vi "Instrument.MessageFromProcess.vi"(6 "Message ID":u32, 8 "error in (no error)":errorcluster, 9 "Message.Data":variant, 10 "Message.Command":string, 11 "Instrument":refnum<class "Instrument.lvclass">) -> (0 "error out":errorcluster, 3 "Instrument out":refnum<class "Instrument.lvclass">)   [LabVIEW 2016, in "Instrument.lvclass"]
doc: "---------------------------------------------------------------\nJKI State Machine Objects™\nhttp://jki.net/state-machine-objects/\nCopyright (C) 2005-2015, JKI <info@jki.net>\nALL RIGHTS RESERVEDJKI State Machine Objects (SMO) 1.0.0.4\nJKI - JKI\nCopyright (c) 2015, JKI"
uses:
  Instrument.lvclass
  Typedefs/PublicEvents--Instrument.MessageFromProcess.ctl
  Instrument.lvclass/Instrument.ctl
panel:
  # "For instructions on how to use the JKI State Machine Objects, examples and video tutorials, visit:\nhttp://jki.net/state-machine-objects/\n\nJKI State Machine Objects™\nhttp://jki.net/state-machine-objects/\nCopyright (C) 2005-2015, JKI <info@jki.net>\nALL RIGHTS RESERVED"
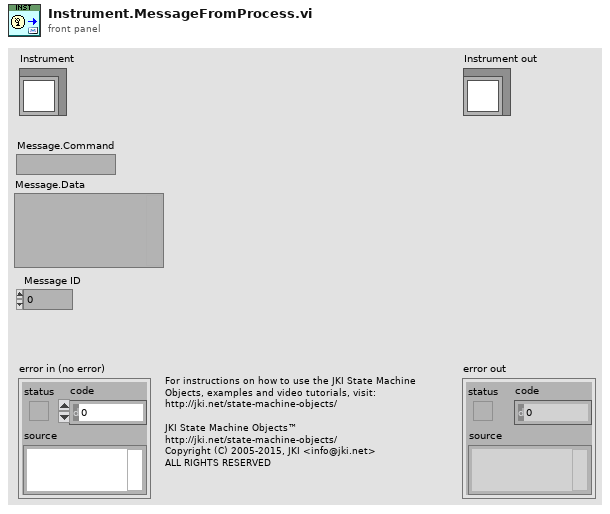
[diagram p1: front panel]
types:
  T1 = typedef "Instrument.lvclass/PublicEvents--Instrument.MessageFromProcess.ctl" = cluster{"Message":cluster{"Command":string, "Data":variant}, "Message ID":u32}
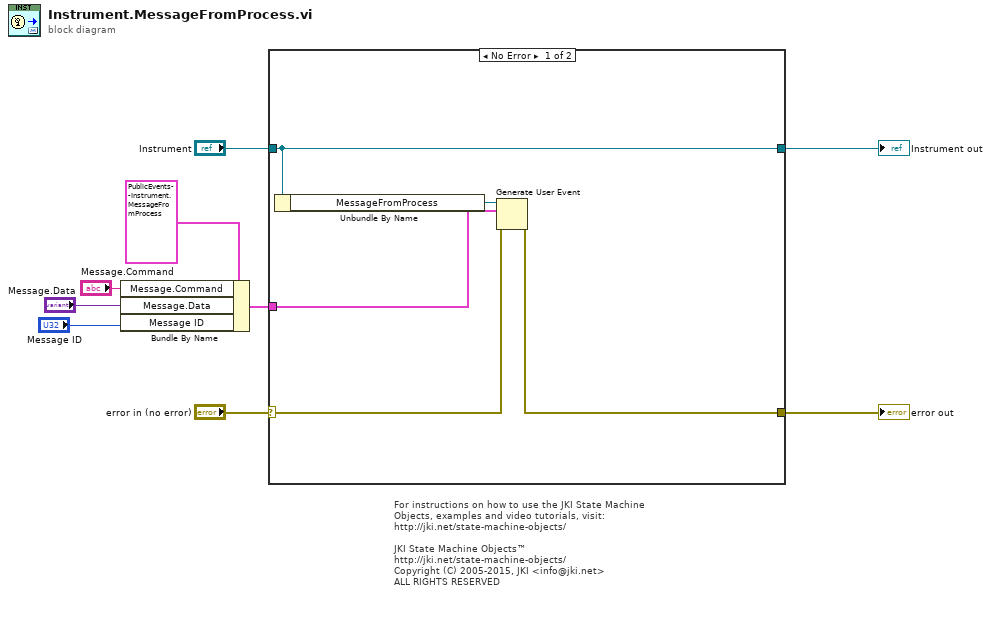
[diagram p0: block diagram]
diagram:
  # "For instructions on how to use the JKI State Machine Objects, examples and video tutorials, visit:\nhttp://jki.net/state-machine-objects/\n\nJKI State Machine Objects™\nhttp://jki.net/state-machine-objects/\nCopyright (C) 2005-2015, JKI <info@jki.net>\nALL RIGHTS RESERVED"
  n1 = Bundle By Name(cluster=T1 {"Message"={"Command"="", "Data"=variant(bool FALSE)}, "Message ID"=0} ("MessageFromProcess"), "Message.Command"="Message.Command", "Message.Data"="Message.Data", "Message ID"="Message ID") -> (w4:T1)
  n2 = case shown="No Error" "error in (no error)" {
    selector: "error in (no error)" -> [w14 w16]
    tunnel: [w11 w16] -> w8
    tunnel: [w10 w15] -> w9
    tunnel: "Instrument" -> [w10 w15]
    tunnel: w4 -> [w13 _]
    frame No Error {
      n3 = Unbundle By Name(w10) -> ("MessageFromProcess"=w12:refnum<user-event>)
      n4 = Generate User Event(user event=w12, event data cluster=w13, error in=w14) -> (error out=w11:errorcluster)  [unwired: 1 in, 1 out]
    }
    frame Error {
    }
  }
  "error out" <- w8
  "Instrument out" <- w9
